vi "Fetch Waveform.vi"(0 "VISA resource name":refnum<visa-resource-name>, 5 "Channel (0:Channel1)":u16(ring) items=["Channel1", "Channel2", "Channel3", "Channel4", "Math1", "Math2", "Math3", "Math3", "Reference1", "Reference2", "Reference3", "Reference4"], 9 "Maximum Time (10000ms)":u32=10000, 11 "error in (no error)":errorcluster) -> (4 "VISA resource name out":refnum<visa-resource-name>, 6 "Waveform Data":waveform(dbl)(graph)={"t0"=timestamp(3.694502999999883e-07 s since 1904-01-01), "dt"=5e-07, "Y"=array[10000 elements]}, 12 "t0":timestamp, 13 "dt":dbl, 14 "raw array data":dbl[](array[numeric]), 15 "error out":errorcluster)   [LabVIEW 2011]
doc: "Returns the waveform that an oscilloscope acquires for a channel you specify. An acquisition that you initiate before calling this VI generates the waveform.\n\nYou first enable channels with the Configure Channel VI. Then you use the Initiate VI to start an acquisition on the enabled channels. An oscilloscope concurrently acquires waveforms for these channels. You must call the Fetch Waveform VI separately to obtain waveforms for each enabled channel. However, you also can call the Read Waveform VI instead of using the above low-level VIs.\n\n<B>Note:</B> Use the Fetch Waveform VI only with other low-level VIs, such as the Initiate VI, the Abort VI, and the Fetch Waveform Measurement VI. High-level VIs such as the Read Waveform VI automatically incorporate the functions of the Initiate VI and the Fetch Waveform VI. The Fetch Waveform VI does not check the status of an instrument."
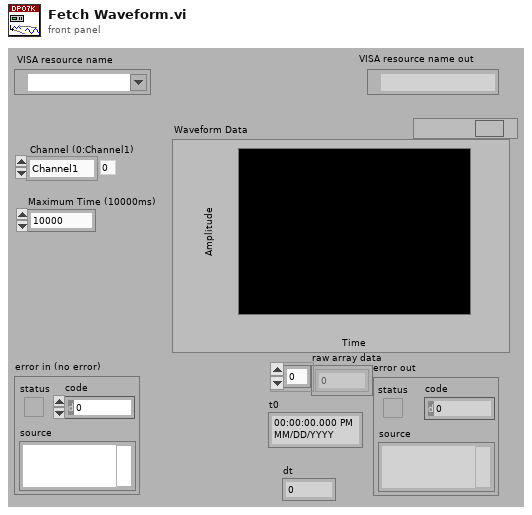
[diagram p1: front panel]
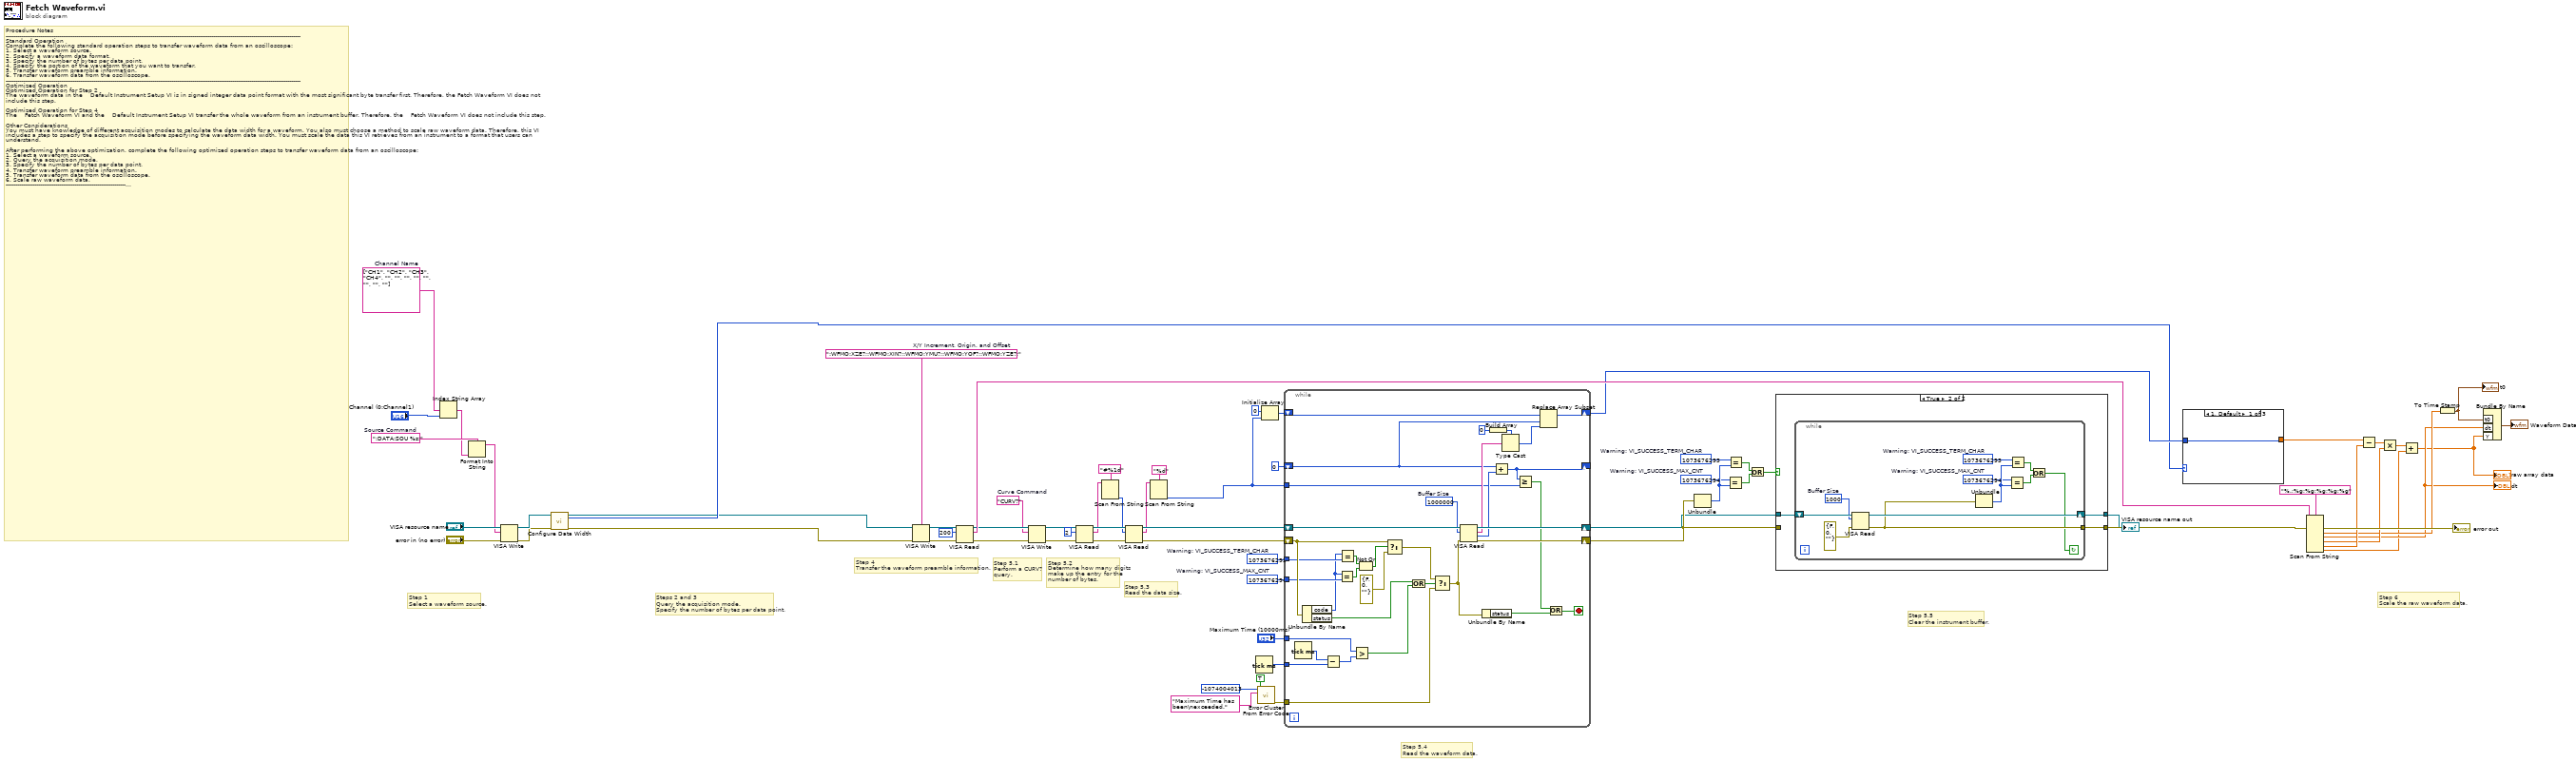
[diagram p0: block diagram]
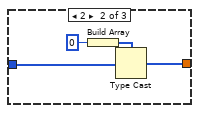
[diagram p2: hidden frame]
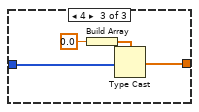
[diagram p3: hidden frame]
diagram:
  w11 = "CURV?"  # Curve Command
  w42 = string[] ["CH1", "CH2", "CH3", "CH4", "", "", "", "", "", "", "", ""]  # Channel Name
  w48 = 1073676294  # Warning: VI_SUCCESS_MAX_CNT
  w49 = 1073676293  # Warning: VI_SUCCESS_TERM_CHAR
  w52 = 1073676294  # Warning: VI_SUCCESS_MAX_CNT
  w51 = 1073676293  # Warning: VI_SUCCESS_TERM_CHAR
  w68 = ":DATA:SOU %s;"  # Source Command
  w37 = ":WFMO:XZE?;:WFMO:XIN?;:WFMO:YMU?;:WFMO:YOF?;:WFMO:YZE?;"  # X/Y Increment, Origin, and Offset
  # "Step 1       \nSelect a waveform source."
  # "Steps 2 and 3\nQuery the acquisition mode. \nSpecify the number of bytes per data point."
  # "Step 6    \nScale the raw waveform data."
  # "Step 5.5    \nClear the instrument buffer."
  # "Step 5.4   \nRead the waveform data."
  # "Step 5.3      \nRead the data size."
  # "Step 5.2      \nDetermine how many digits\nmake up the entry for the \nnumber of bytes."
  # "Step 5.1      \nPerform a CURV?\nquery."
  # "Step 4\nTransfer the waveform preamble information."
  # "Procedure Notes\n-----------------------------------------------------------------------------------------------------------------------------------------------------------\nStandard Operation\nComplete the following standard operation steps to transfer waveform data from an oscilloscope:\n1. Select a waveform source.\n2. Specify a waveform data format.\n3. Specify the number of bytes per data point.\n4. Specify the portion of the waveform that you want to transfer.\n5. Transfer waveform preamble information.\n6. Transfer waveform data from the oscilloscope.\n-----------------------------------------------------------------------------------------------------------------------------------------------------------\nOptimized Operation\nOptimized Operation for Step 2\nThe waveform data in the    Default Instrument Setup VI is in signed integer data point format with the most significant byte transfer first. Therefore, the Fetch Waveform VI does not include this step.\n\nOptimized Operation for Step 4 \nThe    Fetch Waveform VI and the    Default Instrument Setup VI transfer the whole waveform from an instrument buffer. Therefore, the    Fetch Waveform VI does not include this step.\n\nOther Considerations\nYou must have knowledge of different acquisition modes to calculate the data width for a waveform. You also must choose a method to scale raw waveform data. Therefore, this VI includes a step to specify the acquisition mode before specifying the waveform data width. You must scale the data this VI retrieves from an instrument to a format that users can understand.\n\nAfter performing the above optimization, complete the following optimized operation steps to transfer waveform data from an oscilloscope:\n1. Select a waveform source.\n2. Query the acquisition mode.\n3. Specify the number of bytes per data point.\n4. Transfer waveform preamble information.\n5. Transfer waveform data from the oscilloscope.\n6. Scale raw waveform data.\n-----------------------------------------------------------------------------------------------------------------------------------------------------------\nDetailed Steps\nThe following steps detail the behavior of this VI:\n1. Select a waveform source. \n2. Query and determine the acquisition mode. A correct determination is critical to steps 3 and 6.\n    -----------------------------------------------\n    Acquisition Mode |  Data Width   \n    -----------------------------------------------\n    Normal                       |   1                      \n    -----------------------------------------------\n    Peak Detect               |   1                      \n    -----------------------------------------------\n    Hi Res                        |   2                      \n    -----------------------------------------------\n    Envelope                   |   1                      \n    ----------------------------------------------- \n    Average                    |   2                      \n    -----------------------------------------------\n3. Specify the number of bytes per data point. For the Hi Res or Average acquisition modes, set the data width to 2. For all other acquisition modes, set the data width to 1.\n4. Transfer the waveform preamble information. Necessary preamble information includes XZero, XIncrement, YMultiplier, YOffset, and YZero. This VI uses XZero and XIncrement to configure the x-axis of output waveforms and uses YMultiplier, YOffset, and YZero to scale data values. This VI then parses the return string of the preamble query in step 6.\n5. Transfer waveform data from the oscilloscope.\n    5.1 Perform a CURV? query.\n    5.2 Determine how many digits make up the entry for the number of bytes.\n    5.3 Read the data size.\n    5.4 Call the VISA Read VI repeatedly with a buffer size of 10000 until you obtain as much data as the data size specifies. Use      an 8-bit array to store the raw waveform data you obtain. \n    5.5 Continue reading the data remaining in the instrument buffer until the buffer is empty.\n6. Scale the raw waveform data.\n    6.1 Cast the waveform data to a 16-bit array if the data width is 2. Split the waveform data into a minimum and a maximum data array if the acquisition mode is Peak Detect or Envelope. This VI skips this step if the data width is 1.\n    6.2 Parse the preamble information.\n    6.3 Scale the waveform data according to the following formula:\n          Data_Value_in_units = (Raw_Data_Value - YOffset) * YMultiplier + YZero\n          The resulting waveform data has a unit of volts.\n    6.4 Build a waveform graph."
  n1 = Index String Array(1:"Channel (0:Channel1)", 2:w42) -> (0:w67:string)  [unwired: 1 in]
  n2 = Format Into String(format string=w68, w67) -> (resulting string=w39:string)  [unwired: 2 in, 1 out]
  n3 = VISA Write(VISA resource name="VISA resource name", write buffer=w39, error in (no error)="error in (no error)") -> (VISA resource name out=w31:refnum<visa-resource-name>, error out=w30:errorcluster)  [unwired: 1 out]
  n4 = call "Configure Data Width.vi"("error in (no error)"=w30, "VISA resource name"=w31) -> ("error out"=w12:errorcluster, "Width"=w16:i32, "VISA resource name out"=w13:refnum<visa-resource-name>)  [unwired: 7 in]
  n5 = VISA Write(VISA resource name=w13, write buffer=w37, error in (no error)=w12) -> (VISA resource name out=w65:refnum<visa-resource-name>, error out=w64:errorcluster)  [unwired: 1 out]
  n6 = VISA Read(VISA resource name=w65, byte count=u32 200, error in (no error)=w64) -> (VISA resource name out=w29:refnum<visa-resource-name>, read buffer=w63:string, error out=w28:errorcluster)  [unwired: 1 out]
  n7 = VISA Write(VISA resource name=w29, write buffer=w11, error in (no error)=w28) -> (VISA resource name out=w1:refnum<visa-resource-name>, error out=w10:errorcluster)  [unwired: 1 out]
  n8 = VISA Read(VISA resource name=w1, byte count=u32 2, error in (no error)=w10) -> (VISA resource name out=w7:refnum<visa-resource-name>, read buffer=w5:string, error out=w6:errorcluster)  [unwired: 1 out]
  n9 = Scan From String(format string="#%1d", input string=w5) -> (output 1=w4:i32)  [unwired: 3 in, 3 out]
  n10 = VISA Read(VISA resource name=w7, byte count=w4, error in (no error)=w6) -> (VISA resource name out=w27:refnum<visa-resource-name>, read buffer=w2:string, error out=w26:errorcluster)  [unwired: 1 out]
  n11 = Scan From String(format string="%d", input string=w2) -> (output 1=w59:i32)  [unwired: 3 in, 3 out]
  n12 = Tick Count (ms)() -> (millisecond timer value=w19:u32)
  n13 = call <vilib>:"Error Cluster From Error Code.vi"("show call chain? (False)"=TRUE, "error message (\"\")"="Maximum Time has been\nexceeded." ("error message (\"\")"), "error code (0)"=-1074004013) -> ("error out"=w17:errorcluster)  [unwired: 6 in]
  n14 = Initialize Array(i8 0 ("element"), w59) -> (w57:i8[])
  n15 = while {
    shift-right: [w101] -> w14
    shift-left: w27 -> [w103]
    shift-right: [w100] -> w15
    shift-left: w26 -> [w89]
    shift-right: [w96] -> w47
    shift-left: w57 -> [w97]
    tunnel: w59 -> [w93]
    shift-right: [w90] -> _
    shift-left: 0 -> [w91]
    tunnel: w49 -> [w88]
    tunnel: w48 -> [w87]
    tunnel: w19 -> [w81]
    tunnel: "Maximum Time (10000ms)" -> [w80]
    tunnel: w17 -> [w75]
    stop <- w71 stop-if-true
    w102 = 1000000  # Buffer Size
    n16 = Tick Count (ms)() -> (millisecond timer value=w82:u32)
    n17 = Unbundle By Name(w89) -> ("code"=w86:i32, "status"=w74:bool)
    n18 = Subtract(x=w82, y=w81) -> (x-y=w79:u32)
    n19 = Equal?(x=w86, y=w87) -> (x = y?=w84:bool)
    n20 = Equal?(x=w86, y=w88) -> (x = y?=w85:bool)
    n21 = Greater?(x=w80, y=w79) -> (0:w73:bool)
    n22 = Not Or(1:w84, 2:w85) -> (0:w83:bool)
    n23 = Select(t=w89, s=w83, f=errorcluster {"status"=FALSE, "code"=0, "source"=""} ("error in (no error)")) -> (s? t:f=w76:errorcluster)
    n24 = Or(x=w74, y=w73) -> (x .or. y?=w77:bool)
    n25 = Select(t=w76, s=w77, f=w75) -> (s? t:f=w70:errorcluster)
    n26 = VISA Read(VISA resource name=w103, byte count=w102, error in (no error)=w70) -> (VISA resource name out=w101:refnum<visa-resource-name>, read buffer=w95:string, return count=w94:u32, error out=w100:errorcluster)
    n27 = Unbundle By Name(w70) -> ("status"=w69:bool)
    n28 = Build Array(i8 0) -> (w99:i8[])
    n29 = Add(x=w91, y=w94) -> (x+y=w90:u32)
    n30 = Type Cast(type=w99, x=w95) -> (*(type *) &x=w92:i8[])
    n31 = Greater Or Equal?(x=w90, y=w93) -> (x >= y?=w72:bool)
    n32 = Replace Array Subset(array=w97, new element=w92, index=w91) -> (w96:i8[])
    n33 = Or(x=w72, y=w69) -> (x .or. y?=w71:bool)
  }
  n34 = Unbundle(w15) -> ("code"=w53:i32)  [unwired: 2 out]
  n35 = Equal?(x=w52, y=w53) -> (x = y?=w55:bool)
  n36 = Equal?(x=w51, y=w53) -> (x = y?=w56:bool)
  n37 = Or(x=w56, y=w55) -> (x .or. y?=w54:bool)
  n38 = case shown="True" w54 {
    tunnel: w14 -> [w105 w108]
    tunnel: w15 -> [w104 _]
    tunnel: [w105 w107] -> w60
    tunnel: [w104 w106] -> w62
    frame False {
    }
    frame True {
      n39 = while {
        shift-right: [w118] -> w107
        shift-left: w108 -> [w119]
        tunnel: [w111] -> w106
        stop <- w110 continue-if-true
        w113 = 1073676294  # Warning: VI_SUCCESS_MAX_CNT
        w112 = 1073676293  # Warning: VI_SUCCESS_TERM_CHAR
        w117 = u32 1000  # Buffer Size
        n40 = VISA Read(VISA resource name=w119, byte count=w117, error in (no error)=errorcluster {"status"=FALSE, "code"=0, "source"=""}) -> (VISA resource name out=w118:refnum<visa-resource-name>, error out=w111:errorcluster)  [unwired: 2 out]
        n41 = Unbundle(w111) -> ("code"=w114:i32)  [unwired: 2 out]
        n42 = Equal?(x=w113, y=w114) -> (x = y?=w115:bool)
        n43 = Equal?(x=w112, y=w114) -> (x = y?=w116:bool)
        n44 = Or(x=w116, y=w115) -> (x .or. y?=w110:bool)
      }
    }
  }
  "VISA resource name out" <- w60
  n45 = case shown="1, Default" w16 {
    tunnel: w47 -> [w120 w122 w126]
    tunnel: [w120 w121 w125] -> w35
    frame 1, Default {
    }
    frame 2 {
      n46 = Build Array(i16 0 ("element")) -> (w123:i16[])
      n47 = Type Cast(type=w123, x=w122) -> (*(type *) &x=w121:i16[])
    }
    frame 4 {
      n48 = Build Array(sgl 0.0 ("element")) -> (w127:sgl[])
      n49 = Type Cast(type=w127, x=w126) -> (*(type *) &x=w125:sgl[])
    }
  }
  n50 = Scan From String(format string="%.;%g;%g;%g;%g;%g", input string=w63, error in=w62) -> (error out=→"error out":errorcluster, output 1=w34:dbl, output 2=w32:dbl, output 3=w43:dbl, output 4=w44:dbl, output 5=w24:dbl)  [unwired: 6 in, 2 out]
  "dt" <- w32
  n51 = Subtract(x=w35, y=w44) -> (x-y=w45:dbl[])
  n52 = Multiply(x=w45, y=w43) -> (x*y=w25:dbl[])
  n53 = Add(x=w25, y=w24) -> (x+y=w23:dbl[])
  "raw array data" <- w23
  n54 = To Time Stamp(1:w34) -> (0:w33:timestamp)
  "t0" <- w33
  n55 = Bundle By Name ("Build Waveform")("t0"=w33, "dt"=w32, "Y"=w23) -> (→"Waveform Data":waveform(dbl))  [unwired: 1 in]
